vi "Create Message Accessor.vi"(8 "error in (no error)":errorcluster, 10 "Message Metadata":T1, 11 "Server class in":refnum<vi>) -> (0 "error out":errorcluster, 3 "Server class out":refnum<vi>)   [LabVIEW 2019, in "gRPC Scripting Tools.lvlib"]
uses:
  gRPC Scripting Tools.lvlib
  TypeDefs/Message Metadata (Scripting).ctl
  TypeDefs/Message Element Metadata (Scripting).ctl
  TypeDefs/Message Element Type.ctl
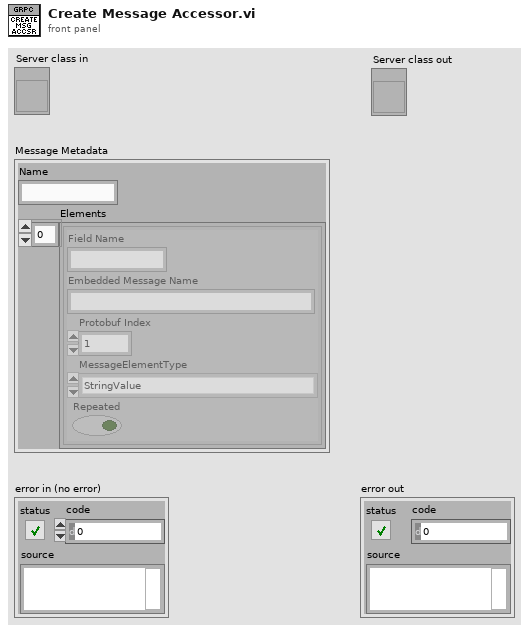
[diagram p1: front panel]
types:
  T1 = typedef "gRPC Scripting Tools.lvlib/Message Metadata (Scripting).ctl" = cluster{"Name":string, "Elements":T2[]}
  T2 = typedef "gRPC Scripting Tools.lvlib/Message Element Metadata (Scripting).ctl" = cluster{"Field Name":string, "Embedded Message Name":string, "Protobuf Index":i32, "MessageElementType":T3, "Repeated":bool}
  T3 = typedef "gRPC Scripting Tools.lvlib/Message Element Type.ctl" = enum32{"Int32Value", "FloatValue", "DoubleValue", "BoolValue", "StringValue", "MessageValue", ""}
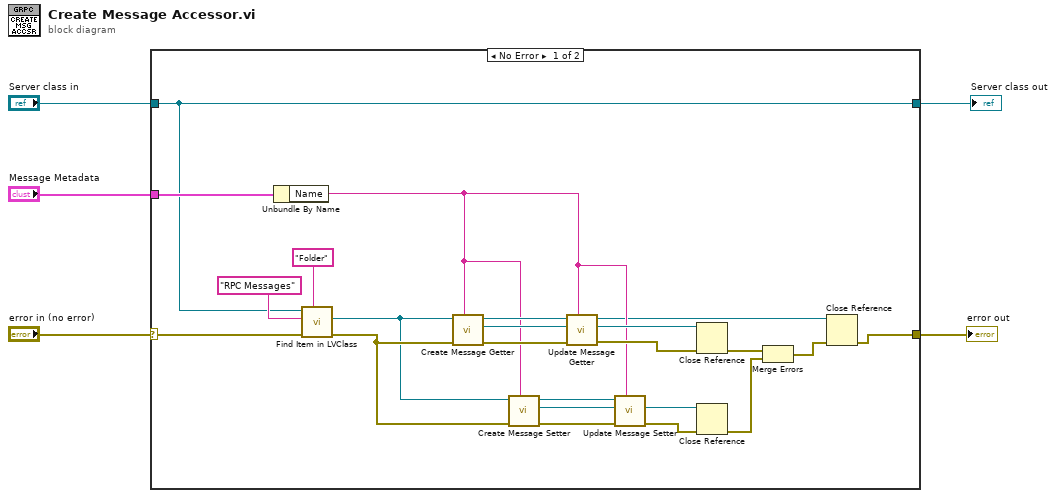
[diagram p0: block diagram]
diagram:
  n1 = case shown="No Error" "error in (no error)" {
    selector: "error in (no error)" -> [w7 w29]
    tunnel: "Server class in" -> [w6 w30]
    tunnel: "Message Metadata" -> [w28 _]
    tunnel: [w8 w29] -> w3
    tunnel: [w6 w30] -> w1
    frame No Error {
      n2 = Unbundle By Name(w28) -> ("Name"=w14:string)
      n3 = call "Find Item in LVClass.vi"("Item Type"="Folder", "error in (no error)"=w7, "Item Name"="RPC Messages", "Class Item in"=w6) -> ("error out"=w20:errorcluster, "Project Item (Class Item)"=w19:refnum<vi>)  [unwired: 4 in, 2 out]
      n4 = call "Create Message Getter.vi"("RPC Message Name"=w14, "error in (no error)"=w20, "RPC Messages Folder (ProjectItem) in"=w19) -> ("error out"=w23:errorcluster, "Message Getter out"=w24:refnum<vi>, "RPC Messages Folder (ProjectItem) out"=w25:refnum<vi>)  [unwired: 6 in]
      n5 = call "Create Message Setter.vi"("RPC Message Name"=w14, "error in (no error)"=w20, "RPC Messages Folder (ProjectItem) in"=w19) -> ("error out"=w18:errorcluster, "Message Setter out"=w16:refnum<vi>, "RPC Messages Folder (ProjectItem) out"=w17:refnum<vi>)  [unwired: 6 in]
      n6 = call "Update Message Getter.vi"("RPC Message Name"=w14, "error in (no error)"=w23, "Message Getter in"=w24, "RPC Messages Folder (ProjectItem) in"=w25) -> ("error out"=w21:errorcluster, "Message Getter out"=w22:refnum<vi>, "RPC Messages Folder (ProjectItem) out"=w10:refnum<vi>)  [unwired: 5 in]
      n7 = call "Update Message Setter.vi"("RPC Message Name"=w14, "error in (no error)"=w18, "Message Getter in"=w16, "RPC Messages Folder (ProjectItem) in"=w17) -> ("error out"=w15:errorcluster, "Message Getter out"=w11:refnum<vi>)  [unwired: 5 in, 1 out]
      n8 = Close Reference(reference=w22, error in (no error)=w21) -> (error out=w13:errorcluster)
      n9 = Close Reference(reference=w11, error in (no error)=w15) -> (error out=w12:errorcluster)
      n10 = Merge Errors(w13, w12) -> (w9:errorcluster)
      n11 = Close Reference(reference=w10, error in (no error)=w9) -> (error out=w8:errorcluster)
    }
    frame Error {
    }
  }
  "error out" <- w3
  "Server class out" <- w1
